vi "Save_Image.vi"(4 "Image Quality":u32=750 max=1000 step=10, 6 "Save Format":enum16{"JPEG", "PNG", "BMP"}(ring), 8 "error in (no error)":errorcluster, 10 "Dest Path":path, 11 "Refnum in":T1) -> (0 "error out":errorcluster, 3 "Refnum out":T1)   [LabVIEW 2020]
uses:
  <vilib>/vision/Image Controls.llb/IMAQ Image.ctl
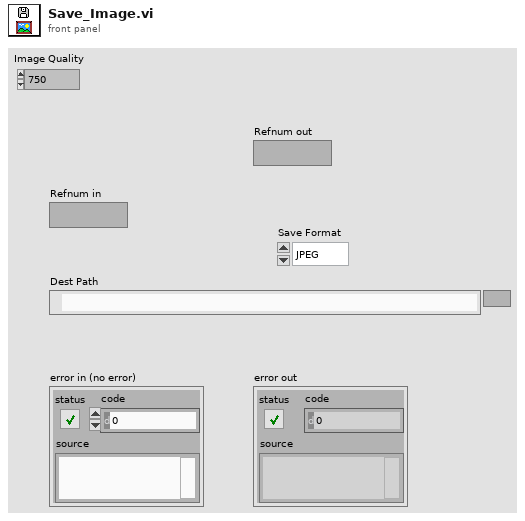
[diagram p1: front panel]
types:
  T1 = typedef "IMAQ Image.ctl" = refnum<image>
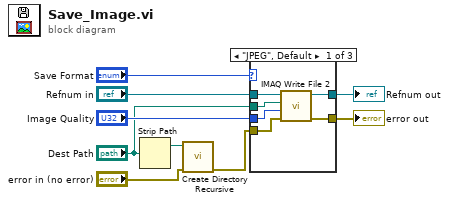
[diagram p0: block diagram]
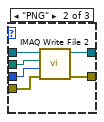
[diagram p2: hidden frame]
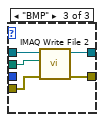
[diagram p3: hidden frame]
diagram:
  n1 = Strip Path(path="Dest Path") -> (stripped path=w1:path)  [unwired: 1 out]
  n2 = call <vilib>:"Create Directory Recursive.vi"("error in (no error)"="error in (no error)", "directory"=w1) -> ("error out"=w3:errorcluster)  [unwired: 3 in, 2 out]
  n3 = case shown="\"JPEG\", Default" "Save Format" {
    tunnel: [w15 w21 w26] -> w9
    tunnel: [w14 w20 w25] -> w8
    tunnel: "Dest Path" -> [w13 w19 w24]
    tunnel: "Refnum in" -> [w12 w18 w23]
    tunnel: w3 -> [w11 w17 w22]
    tunnel: "Image Quality" -> [w10 w16 _]
    frame "JPEG", Default {
      n4 = call-poly "IMAQ Write File 2"("error in (no error)"=w11, "Image Quality"=w10, "File Path"=w13, "Image"=w12) -> ("error out"=w14:errorcluster, "Image Out (duplicate)"=w15:T1)  [unwired: 6 in]
    }
    frame "PNG" {
      n5 = call-poly "IMAQ Write File 2"("error in (no error)"=w17, "Image Quality"=w16, "File Path"=w19, "Image"=w18) -> ("error out"=w20:errorcluster, "Image Out (duplicate)"=w21:T1)  [unwired: 6 in]
    }
    frame "BMP" {
      n6 = call-poly "IMAQ Write File 2"("error in (no error)"=w22, "File Path"=w24, "Image"=w23) -> ("error out"=w25:errorcluster, "Image Out (duplicate)"=w26:T1)  [unwired: 7 in]
    }
  }
  "Refnum out" <- w9
  "error out" <- w8
